vi "bucketOf.vi"(8 "error in (no error)":errorcluster, 10 "Key":string, 11 "HashMap in":refnum<class "HashMap.lvclass">) -> (0 "error out":errorcluster, 2 "Bucket Index":i32, 3 "HashMap out":refnum<class "HashMap.lvclass">)   [LabVIEW 2017, in "HashMap.lvclass"]
uses:
  <userlib>/836-Library/Data_Structures/HashMap/HashMap.lvclass
  <userlib>/836-Library/Data_Structures/HashMap/HashMap.lvclass/HashMap.ctl
  <userlib>/836-Library/Data_Structures/Bucket/Bucket.lvclass
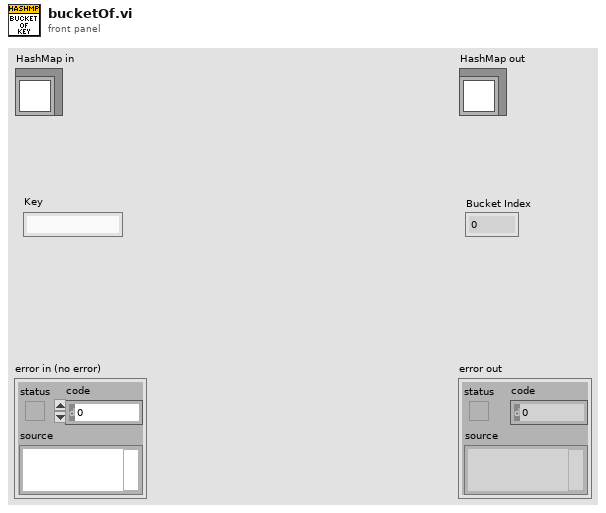
[diagram p1: front panel]
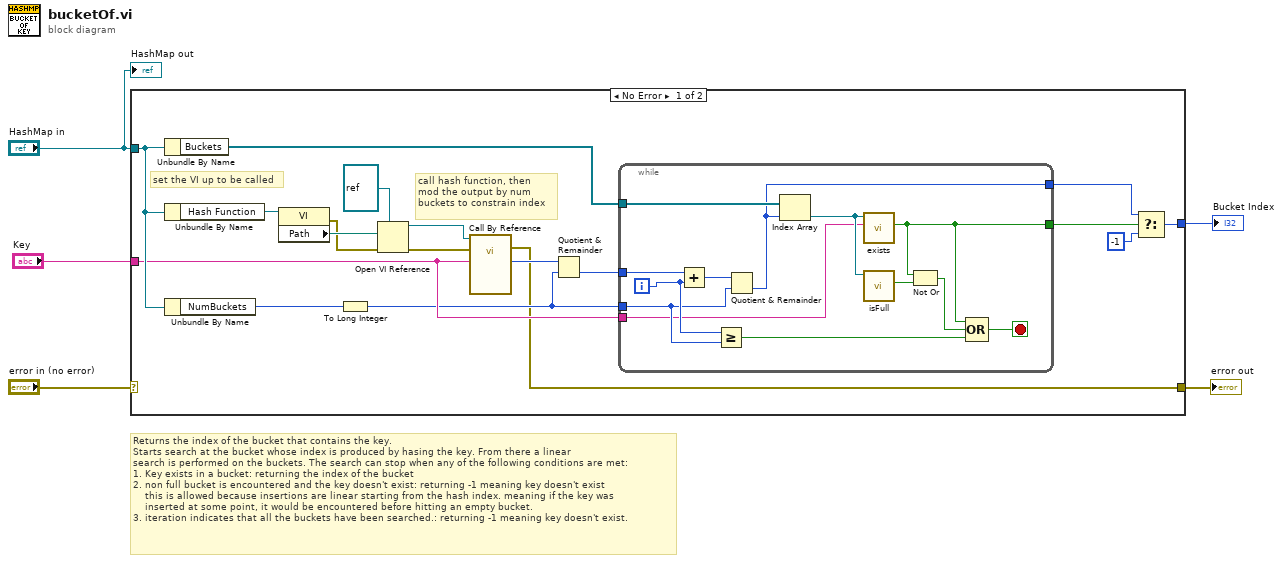
[diagram p0: block diagram]
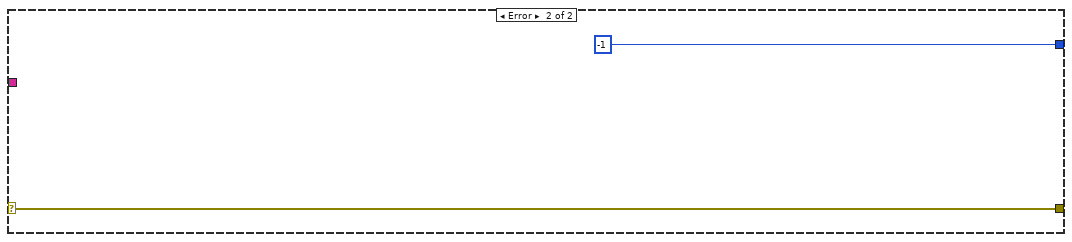
[diagram p2: hidden frame]
diagram:
  # "Returns the index of the bucket that contains the key.\nStarts search at the bucket whose index is produced by hasing the key. From there a linear\nsearch is performed on the buckets. The search can stop when any of the following conditions are met:\n1. Key exists in a bucket: returning the index of the bucket\n2. non full bucket is encountered and the key doesn't exist: returning -1 meaning key doesn't exist\n    this is allowed because insertions are linear starting from the hash index. meaning if the key was\n    inserted at some point, it would be encountered before hitting an empty bucket.\n3. iteration indicates that all the buckets have been searched.: returning -1 meaning key doesn't exist."
  n1 = case shown="No Error" "error in (no error)" {
    selector: "error in (no error)" -> [_ w38]
    tunnel: [w6 w38] -> w4
    tunnel: "HashMap in" -> [w16 _]
    tunnel: "Key" -> [w12 _]
    tunnel: [w7 -1 ("f")] -> w1
    frame No Error {
      # "call hash function, then\nmod the output by num\nbuckets to constrain index"
      # "set the VI up to be called"
      n2 = Unbundle By Name(w16) -> ("Buckets"=w15:refnum<class "Bucket.lvclass">[])
      n3 = Unbundle By Name(w16) -> ("Hash Function"=w23:refnum<vi>)
      n4 = Unbundle By Name(w16) -> ("NumBuckets"=w13:u32)
      n5 = property class="VI"(reference=w23) -> (error out=w19:errorcluster, "Path"=w22:path)  [unwired: 1 in, 1 out]
      n6 = To Long Integer(number=w13) -> (32bit integer=w9:i32)
      n7 = Open VI Reference(type specifier VI Refnum (for type only)=refnum<vi> refnum, vi path=w22, error in (no error)=w19) -> (vi reference=w20:refnum<vi>, error out=w18:errorcluster)  [unwired: 3 in]
      n8 = call-by-ref "?"(reference=w20, error in=w18, "Key"=w12) -> (error out=w6:errorcluster, "Hash"=w17:i32)  [unwired: 10 in, 1 out]
      n9 = Quotient & Remainder(x=w17, y=w9) -> (floor(x/y)=w14:i32)  [unwired: 1 out]
      n10 = while {
        tunnel: w15 -> [w34]
        tunnel: w14 -> [w36]
        tunnel: w9 -> [w32]
        tunnel: w12 -> [w29]
        tunnel: [w26] -> w11
        tunnel: [w25] -> w10
        i -> [w33]
        stop <- w24 stop-if-true
        n11 = Add(x=w36, y=w33) -> (x+y=w35:i32)
        n12 = Greater Or Equal?(x=w33, y=w32) -> (x >= y?=w31:bool)
        n13 = Quotient & Remainder(x=w35, y=w32) -> (floor(x/y)=w25:i32)  [unwired: 1 out]
        n14 = Index Array(array=w34, index=w25) -> (element=w30:refnum<class "Bucket.lvclass">)
        n15 = call <userlib>:"exists.vi"("Key"=w29, "Bucket in"=w30) -> ("Exists?"=w26:bool)  [unwired: 7 in, 2 out]
        n16 = call <userlib>:"isFull.vi"("Bucket in"=w30) -> ("Full?"=w28:bool)  [unwired: 8 in, 2 out]
        n17 = Not Or(1:w28, 2:w26) -> (0:w27:bool)
        n18 = Compound Arithmetic op=OR(w26, w27, w31) -> (w24:bool)
      }
      n19 = Select(t=w10, s=w11, f=-1) -> (s? t:f=w7:i32)
    }
    frame Error {
    }
  }
  "error out" <- w4
  "Bucket Index" <- w1
  "HashMap out" <- "HashMap in"
